vi "Get Default Data from TD__ogtk.vi"(8 "error in (no error)":errorcluster, 10 "Type Descriptor":T1) -> (0 "error out":errorcluster, 2 "Default VData":variant)   [LabVIEW 2009]
doc: "Returns default data of the type defined by the TD. This VI calls itself recursively.\n\nThis VI is <b>Reentrant</b>"
uses:
  Type Descriptor__ogtk.ctl
panel:
  # "Please visit http://www.OpenG.org to learn about the\nOpen Source LabVIEW software movement.\n\nNOTICE -- YOU MUST LEAVE THIS NOTICE IN PLACE.  PER THE TERMS OF THE LICENSE BELOW, YOU MAY SUBLICENSE THIS SOFTWARE \nIN ANY WAY THAT DOES NOT CONFLICT WITH THIS LICENSE.\n\n### BSD License (http://www.opensource.org/licenses/bsd-license.php) Begin ###\n \nCopyright (c) 2002, Jean-Pierre Drolet <drolet_jp@hotmail.com>\nCopyright (c) 2002-2006, Jim Kring <jim@jimkring.com>\nCopyright (c) 2011, Jonathon Green <jg@jgcode.net>\n\nAll rights reserved.\n\nRedistribution and use in source and binary forms, with or without modification, are permitted provided that the following conditions are met:\n\n    * Redistributions of source code must retain the above copyright notice, this list of conditions and the following disclaimer.\n    * Redistributions in binary form must reproduce the above copyright notice, this list of conditions and the following disclaimer in the \n       documentation and/or other materials provided with the distribution.\n    * Neither the name of SciWare, James Kring, Inc., nor the names of its contributors may be used to endorse or promote products derived \n       from this software without specific prior written permission.\n\nTHIS SOFTWARE IS PROVIDED BY THE COPYRIGHT HOLDERS AND CONTRIBUTORS \"AS IS\" AND ANY EXPRESS OR IMPLIED WARRANTIES, \nINCLUDING, BUT NOT LIMITED TO, THE IMPLIED WARRANTIES OF MERCHANTABILITY AND FITNESS FOR A PARTICULAR PURPOSE ARE \nDISCLAIMED. IN NO EVENT SHALL THE COPYRIGHT OWNER OR CONTRIBUTORS BE LIABLE FOR ANY DIRECT, INDIRECT, INCIDENTAL,\n SPECIAL, EXEMPLARY, OR CONSEQUENTIAL DAMAGES (INCLUDING, BUT NOT LIMITED TO, PROCUREMENT OF SUBSTITUTE GOODS OR \nSERVICES; LOSS OF USE, DATA, OR PROFITS; OR BUSINESS INTERRUPTION) HOWEVER CAUSED AND ON ANY THEORY OF LIABILITY, \nWHETHER IN CONTRACT, STRICT LIABILITY, OR TORT (INCLUDING NEGLIGENCE OR OTHERWISE) ARISING IN ANY WAY OUT OF THE USE \nOF THIS SOFTWARE, EVEN IF ADVISED OF THE POSSIBILITY OF SUCH DAMAGE.\n\n### BSD License End ###"
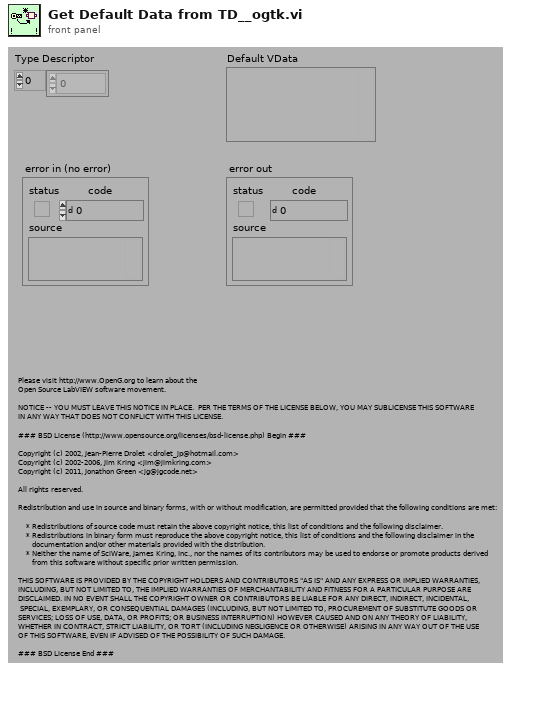
[diagram p1: front panel]
types:
  T1 = typedef "Type Descriptor__ogtk.ctl" = i16[]
  T2 = typedef "Type Descriptor Header__ogtk.ctl" = cluster{"length":u16, "private":u8, "type":T3, "# elements":u16}
  T3 = typedef "Type Descriptor Enumeration__ogtk.ctl" = enum8{"<Null>", "I8", "I16", "I32", "I64", "U8", "U16", "U32", "U64", "SGL", "DBL", "EXT", "CSG", "CDB", "CXT", "0x0F", "0x10", "0x11", "0x12", "0x13", "0x14", "Enum U8", "Enum U16", "Enum U32", "Enum U64", "SGL PQ", "DBL PQ", "EXT PQ", "CSG PQ", "CDB PQ", "CXT PQ", "0x1F", "0x20", "Boolean", "0x22", "0x23", "0x24", "0x25", "0x26", "0x27", "0x28", "0x29", "0x2A", "0x2B", "0x2C", "0x2D", "0x2E", "0x2F", "String", "0x31", "Path", "Pict", "0x34", "0x35", "0x36", "DAQ", "0x38", "0x39", "0x3A", "0x3B", "0x3C", "0x3D", "0x3E", "0x3F", "Array", "0x41", "0x42", "0x43", "0x44", "0x45", "0x46", "0x47", "0x48", "0x49", "0x4A", "0x4B", "0x4C", "0x4D", "0x4E", "0x4F", "Cluster", "0x51", "0x52", "Variant", "Waveform", "0x55", "0x56", "0x57", "0x58", "0x59", "0x5A", "0x5B", "0x5C", "0x5D", "0x5E", "0x5F", "0x60", "0x61", "0x62", "0x63", "0x64", "0x65", "0x66", "0x67", "0x68", "0x69", "0x6A", "0x6B", "0x6C", "0x6D", "0x6E", "0x6F", "Refnum"}
  T4 = typedef "Waveform Subtype Enum__ogtk.ctl" = enum8{"<Not a Waveform Type>", "0x01", "Analog 16-bit signed", "Analog Double-Precision", "0x04", "Analog Single Precision", "Timestamp", "Digital Data", "Digital Waveform", "Dynamic Data", "Analog Extended-Precision", "Analog 8-bit unsigned", "Analog 16-bit unsigned", "Analog 32-bit unsigned", "Analog 8-bit signed", "Analog 32-bit signed", "Analog Complex Single-Precision", "Analog Complex Double-Precision", "Analog Complex Extended Precision", "Analog 64-bit signed", "Analog 64-bit unsigned"}
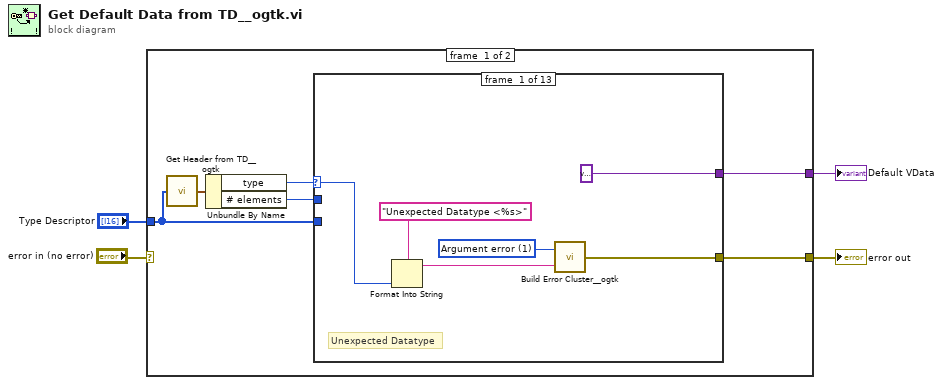
[diagram p0: block diagram]
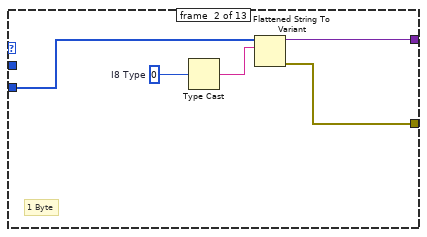
[diagram p2: hidden frame]
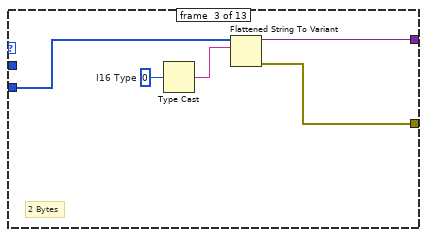
[diagram p3: hidden frame]
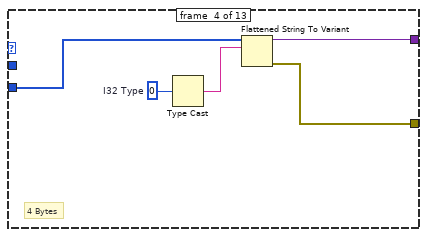
[diagram p4: hidden frame]
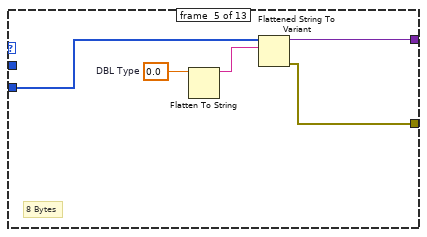
[diagram p5: hidden frame]
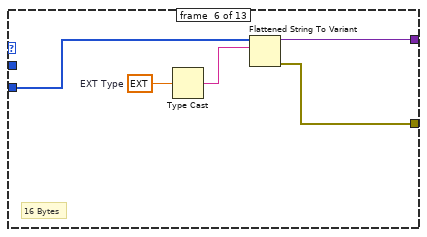
[diagram p6: hidden frame]
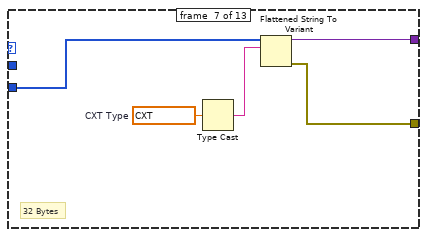
[diagram p7: hidden frame]
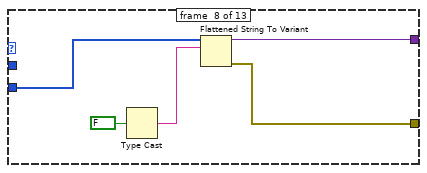
[diagram p8: hidden frame]
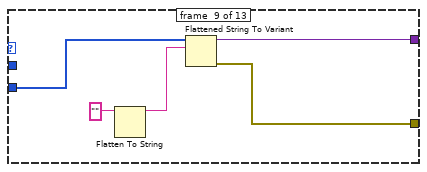
[diagram p9: hidden frame]
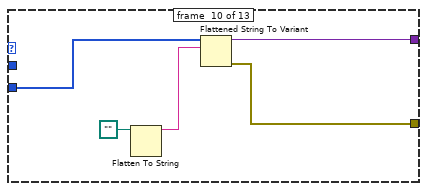
[diagram p10: hidden frame]
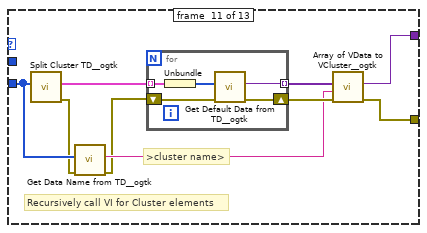
[diagram p11: hidden frame]
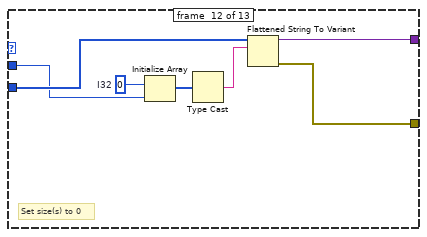
[diagram p12: hidden frame]
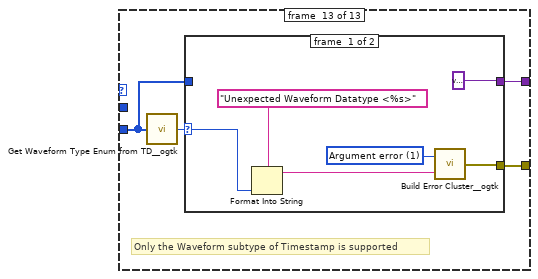
[diagram p13: hidden frame]
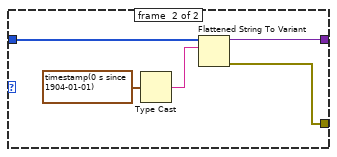
[diagram p14: hidden frame]
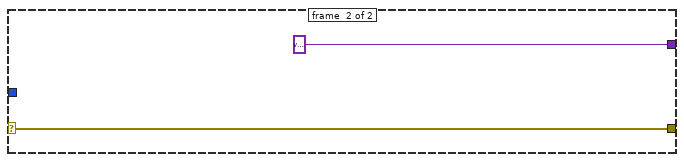
[diagram p15: hidden frame]
diagram:
  n1 = case shown="No Error" "error in (no error)" {
    selector: "error in (no error)" -> [_ w99]
    tunnel: [w10 w99] -> w2
    tunnel: "Type Descriptor" -> [w5 _]
    tunnel: [w9 variant] -> w1
    frame #0 {
      n2 = call "Get Header from TD__ogtk.vi"("Type Descriptor"=w5) -> ("Type Descriptor Header"=w8:T2)
      n3 = Unbundle By Name(w8) -> ("type"=w7:T3, "# elements"=w6:u16)
      n4 = case shown="\"Cluster\"" w7 {
        selector: w7 -> [w13 _ _ _ _ _ _ _ _ _ _ _ _]
        tunnel: [w12 w17 w24 w27 w33 w38 w44 w49 w52 w57 w63 w81 w85] -> w10
        tunnel: w5 -> [_ w19 w25 w29 w34 w40 w43 w50 w54 w60 w67 w80 w84]
        tunnel: [variant w18 w23 w28 w32 w37 w42 w47 w53 w58 w64 w82 w86] -> w9
        tunnel: w6 -> [_ _ _ _ _ _ _ _ _ _ _ w76 _]
        frame #0 {
          w14 = 1 items=["No error", "Argument error", "Memory is full", "Out of zone", "End of file", "File already open", "Generic file I/O error", "File not found", "File permission error", "Disk is full", "Duplicate path", "Too many files open", "System feature not enabled", "Resource file not found", "Cannot add resource", "Resource not found", "Image not found", "Image memory error", "Pen does not exist", "Config type invalid", "Config token not found", "Config parse error", "Config memory error", "Bad external code format", "Bad external code offset", "External code not present", "Null window", "Destroy window error", "Null menu", "Print aborted", "Bad print record", "Print driver error", "Windows error during printing", "Memory error during printing", "Print dialog error", "Generic print error", "Invalid device refnum", "Device not found", "Device parameter error", "Device unit error", "Cannot open device", "Device call aborted", "Generic error", "Cancelled by user", "Object ID too low", "Object ID too high", "Object not in heap", "Unknown heap", "Unknown object (invalid DefProc)", "Unknown object (DefProc not in table)", "Message out of range", "Invalid (null) method", "Unknown message", "Manager call not supported", "Bad address", "Network operation in progress", "Network operation timed out", "Connection is busy", "Network attribute not supported", "Network error", "Address in use", "System out of memory", "Connection aborted", "Connection refused", "Not connected", "Already connected", "Connection closed", "Initialization error (interapplication manager)", "Bad occurrence", "Wait on unbound occurrence handler", "Occurrence queue overflow", "Datalog type conflict", "Unused", "Unrecognized type (interapplication manager)", "Memory corrupt", "Failed to make temporary DLL", "Old CIN version", "Drag socket not found", "Failed to load drop-object", "Failed to register OLE object", "Failed to release OLE object", "Format specifier type mismatch", "Unknown format specifier", "Too few format specifiers", "Too many format specifiers", "Scan failed", "Newer CIN version", "Error converting to variant", "Runtime menu error", "Password tampered", "Variant attribute not found", "Incompatible variant data type", "Event data is not available", "Event Store is not present", "Occurrence is not found", "Event Queue is not created", "Event info is not available", "Refnum passed is NULL", "Error retrieving Class GUID", "Error retrieving CoClass GUID", "Error retrieving TypeLib GUID.", "Bad built application magic bytes.", "Specific driver is different from the specific driver associated with the Logical Name.", "There is no session opened to the class driver.", "Max Error", "MAX - Error with config objects", "MAX - Error loading configuration", "MAX - Group not supported"]
          # "Unexpected Datatype"
          n5 = Format Into String(format string="Unexpected Datatype <%s>" ("Format String"), w13) -> (resulting string=w16:string)  [unwired: 2 in, 1 out]
          n6 = call <userlib>:"Build Error Cluster__ogtk.vi"("String to Prepend to source (\"\")"=w16, "code"=w14) -> ("error out"=w12:errorcluster)
        }
        frame #1 {
          w21 = i8 0  # I8 Type
          # "1 Byte"
          n7 = Type Cast(x=w21) -> (*(type *) &x=w20:string)  [unwired: 1 in]
          n8 = Flattened String To Variant(6:w20, 7:w19) -> (0:w17:errorcluster, 3:w18:variant)  [unwired: 1 in]
        }
        frame #2 {
          w26 = i16 0  # I16 Type
          # "2 Bytes"
          n9 = Type Cast(x=w26) -> (*(type *) &x=w22:string)  [unwired: 1 in]
          n10 = Flattened String To Variant(6:w22, 7:w25) -> (0:w24:errorcluster, 3:w23:variant)  [unwired: 1 in]
        }
        frame #3 {
          w31 = 0  # I32 Type
          # "4 Bytes"
          n11 = Type Cast(x=w31) -> (*(type *) &x=w30:string)  [unwired: 1 in]
          n12 = Flattened String To Variant(6:w30, 7:w29) -> (0:w27:errorcluster, 3:w28:variant)  [unwired: 1 in]
        }
        frame #4 {
          w36 = 0.0  # DBL Type
          # "8 Bytes"
          n13 = Flatten To String(anything=w36) -> (data string=w35:string)  [unwired: 3 in, 2 out]
          n14 = Flattened String To Variant(6:w35, 7:w34) -> (0:w33:errorcluster, 3:w32:variant)  [unwired: 1 in]
        }
        frame #5 {
          w41 = ext 0.0  # EXT Type
          # "16 Bytes"
          n15 = Type Cast(x=w41) -> (*(type *) &x=w39:string)  [unwired: 1 in]
          n16 = Flattened String To Variant(6:w39, 7:w40) -> (0:w38:errorcluster, 3:w37:variant)  [unwired: 1 in]
        }
        frame #6 {
          w46 = cxt 0.0+0.0i  # CXT Type
          # "32 Bytes"
          n17 = Type Cast(x=w46) -> (*(type *) &x=w45:string)  [unwired: 1 in]
          n18 = Flattened String To Variant(6:w45, 7:w43) -> (0:w44:errorcluster, 3:w42:variant)  [unwired: 1 in]
        }
        frame #7 {
          n19 = Type Cast(x=FALSE ("status")) -> (*(type *) &x=w48:string)  [unwired: 1 in]
          n20 = Flattened String To Variant(6:w48, 7:w50) -> (0:w49:errorcluster, 3:w47:variant)  [unwired: 1 in]
        }
        frame #8 {
          n21 = Flatten To String(anything="") -> (data string=w55:string)  [unwired: 3 in, 2 out]
          n22 = Flattened String To Variant(6:w55, 7:w54) -> (0:w52:errorcluster, 3:w53:variant)  [unwired: 1 in]
        }
        frame #9 {
          n23 = Flatten To String(anything=path "") -> (data string=w59:string)  [unwired: 3 in, 2 out]
          n24 = Flattened String To Variant(6:w59, 7:w60) -> (0:w57:errorcluster, 3:w58:variant)  [unwired: 1 in]
        }
        frame #10 {
          # "Recursively call VI for Cluster elements"
          # ">cluster name>"
          n25 = call "Split Cluster TD__ogtk.vi"("Type Descriptor"=w67) -> ("error out"=w66:errorcluster, "Type Descriptors"=w69:cluster{"Type Descriptor":T1}[])  [unwired: 9 in]
          n26 = call "Get Data Name from TD__ogtk.vi"("error in (no error)"=w66, "Type Descriptor"=w67) -> ("error"=w62:errorcluster, "name"=w65:string)  [unwired: 8 in]
          n27 = for {
            tunnel: w69 -> [w75] mode=indexing
            shift-right: [w72] -> w68
            shift-left: w62 -> [w74]
            tunnel: [w71] -> w70 mode=indexing
            n28 = Unbundle(w75) -> ("Type Descriptor"=w73:T1)
            n29 = call "Get Default Data from TD__ogtk.vi"("error in (no error)"=w74, "Type Descriptor"=w73) -> ("error out"=w72:errorcluster, "Default VData"=w71:variant)  [unwired: 8 in]
          }
          n30 = call "Array of VData to VCluster__ogtk.vi"("error in (no error)"=w68, "Cluster Name"=w65, "Array"=w70) -> ("error out"=w63:errorcluster, "VCluster"=w64:variant)  [unwired: 7 in]
        }
        frame #11 {
          w79 = 0  # I32
          # "Set size(s) to 0"
          n31 = Initialize Array(w79, w76) -> (w78:i32[])
          n32 = Type Cast(x=w78) -> (*(type *) &x=w77:string)  [unwired: 1 in]
          n33 = Flattened String To Variant(6:w77, 7:w80) -> (0:w81:errorcluster, 3:w82:variant)  [unwired: 1 in]
        }
        frame #12 {
          # "Only the Waveform subtype of Timestamp is supported"
          n34 = call "Get Waveform Type Enum from TD__ogtk.vi"("Type Descriptor"=w84) -> ("Waveform Subtype Enum"=w83:T4)  [unwired: 4 in]
          n35 = case shown="Default" w83 {
            selector: w83 -> [w87 _]
            tunnel: [variant w97] -> w86
            tunnel: [w88 w96] -> w85
            tunnel: w84 -> [_ w94]
            frame #0 {
              w90 = 1 items=["No error", "Argument error", "Memory is full", "Out of zone", "End of file", "File already open", "Generic file I/O error", "File not found", "File permission error", "Disk is full", "Duplicate path", "Too many files open", "System feature not enabled", "Resource file not found", "Cannot add resource", "Resource not found", "Image not found", "Image memory error", "Pen does not exist", "Config type invalid", "Config token not found", "Config parse error", "Config memory error", "Bad external code format", "Bad external code offset", "External code not present", "Null window", "Destroy window error", "Null menu", "Print aborted", "Bad print record", "Print driver error", "Windows error during printing", "Memory error during printing", "Print dialog error", "Generic print error", "Invalid device refnum", "Device not found", "Device parameter error", "Device unit error", "Cannot open device", "Device call aborted", "Generic error", "Cancelled by user", "Object ID too low", "Object ID too high", "Object not in heap", "Unknown heap", "Unknown object (invalid DefProc)", "Unknown object (DefProc not in table)", "Message out of range", "Invalid (null) method", "Unknown message", "Manager call not supported", "Bad address", "Network operation in progress", "Network operation timed out", "Connection is busy", "Network attribute not supported", "Network error", "Address in use", "System out of memory", "Connection aborted", "Connection refused", "Not connected", "Already connected", "Connection closed", "Initialization error (interapplication manager)", "Bad occurrence", "Wait on unbound occurrence handler", "Occurrence queue overflow", "Datalog type conflict", "Unused", "Unrecognized type (interapplication manager)", "Memory corrupt", "Failed to make temporary DLL", "Old CIN version", "Drag socket not found", "Failed to load drop-object", "Failed to register OLE object", "Failed to release OLE object", "Format specifier type mismatch", "Unknown format specifier", "Too few format specifiers", "Too many format specifiers", "Scan failed", "Newer CIN version", "Error converting to variant", "Runtime menu error", "Password tampered", "Variant attribute not found", "Incompatible variant data type", "Event data is not available", "Event Store is not present", "Occurrence is not found", "Event Queue is not created", "Event info is not available", "Refnum passed is NULL", "Error retrieving Class GUID", "Error retrieving CoClass GUID", "Error retrieving TypeLib GUID.", "Bad built application magic bytes.", "Specific driver is different from the specific driver associated with the Logical Name.", "There is no session opened to the class driver.", "Max Error", "MAX - Error with config objects", "MAX - Error loading configuration", "MAX - Group not supported"]
              n36 = Format Into String(format string="Unexpected Waveform Datatype <%s>" ("Format String"), w87) -> (resulting string=w92:string)  [unwired: 2 in, 1 out]
              n37 = call <userlib>:"Build Error Cluster__ogtk.vi"("String to Prepend to source (\"\")"=w92, "code"=w90) -> ("error out"=w88:errorcluster)
            }
            frame #1 {
              n38 = Type Cast(x=timestamp(0 s since 1904-01-01) ("Time Stamp")) -> (*(type *) &x=w95:string)  [unwired: 1 in]
              n39 = Flattened String To Variant(6:w95, 7:w94) -> (0:w96:errorcluster, 3:w97:variant)  [unwired: 1 in]
            }
          }
        }
      }
    }
    frame #1 {
    }
  }
  "error out" <- w2
  "Default VData" <- w1
